vi "EXAshminitFlags.vi"(8 "error in (no error)":errorcluster) -> (0 "error out":errorcluster)   [LabVIEW 2016, in "SALLV_EXA.lvlib"]
doc: "void EXA_shm_initFlags();"
uses:
  SALLV_EXA.lvlib
  SALLV_EXA.so
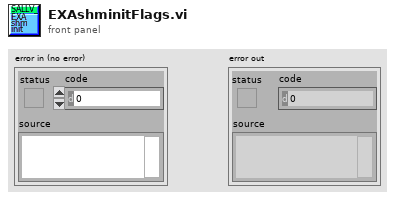
[diagram p1: front panel]
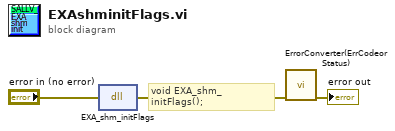
[diagram p0: block diagram]
diagram:
  # "void EXA_shm_initFlags();"
  n1 = dll-call lib="home/andres/Desktop/EXA_SAL_LV/SALLV_EXA.*" fn="EXA_shm_initFlags"(error in="error in (no error)") -> (error out=w2:errorcluster)  [unwired: 3 in, 1 out]
  n2 = call "ErrorConverter(ErrCodeorStatus).vi"("error in (no error)"=w2) -> ("error out"=→"error out":errorcluster)  [unwired: 10 in]
